vi "Case Next Frame.vi"(0 "Diagram in":refnum<vi>, 11 "error in (no error)":errorcluster) -> (4 "Selected Diagram":refnum<vi>, 6 "Selector":refnum<vi>, 8 "Inputs":refnum<vi>[](array[refnum]), 15 "error out":errorcluster)   [LabVIEW 2015, in "Scripting.lvlib"]
doc: "Navigates to the next frame of the Case Structure that owns <B>Diagram in</B>, supplying the frame's diagram at <B>Diagram out</B>. The input inside terminals and selector input terminal corresponding the diagram are output."
uses:
  Scripting.lvlib
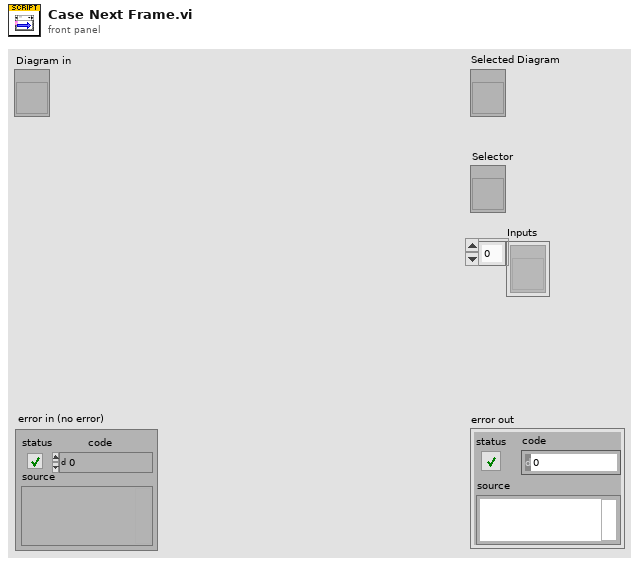
[diagram p1: front panel]
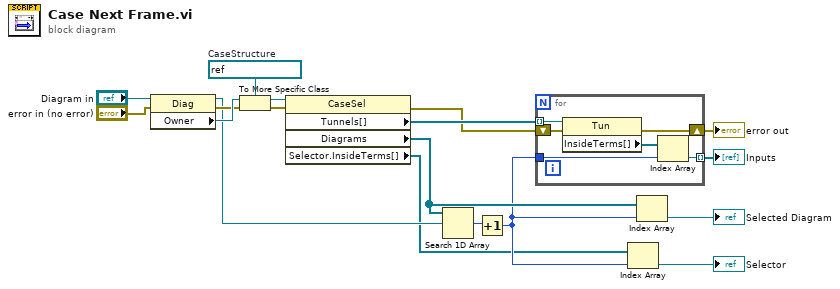
[diagram p0: block diagram]
diagram:
  w17 = refnum<vi> refnum  # CaseStructure
  n1 = property class="Diag"(reference="Diagram in", error in="error in (no error)") -> (reference out=w9:refnum<vi>, error out=w11:errorcluster, "Owner"=w12:refnum<vi>)
  n2 = To More Specific Class(target class=w17, reference=w12, error in=w11) -> (specific class reference=w3:refnum<vi>, error out=w2:errorcluster)
  n3 = property class="CaseSel"(reference=w3, error in=w2) -> (error out=w4:errorcluster, "Tunnels[]"=w5:refnum<vi>[], "Diagrams"=w8:refnum<vi>[], "Selector.InsideTerms[]"=w1:refnum<vi>[])  [unwired: 1 out]
  n4 = Search 1D Array(1D array=w8, element=w9) -> (index of element=w7:i32)  [unwired: 1 in]
  n5 = Increment(x=w7) -> (x+1=w6:i32)
  n6 = for {
    tunnel: w5 -> [w24] mode=indexing
    tunnel: w6 -> [w22]
    shift-right: [w20] -> w16
    shift-left: w4 -> [w21]
    tunnel: [w19] -> w15 mode=indexing
    n7 = property class="Tun"(reference=w24, error in=w21) -> (error out=w20:errorcluster, "InsideTerms[]"=w23:refnum<vi>[])  [unwired: 1 out]
    n8 = Index Array(array=w23, index=w22) -> (element=w19:refnum<vi>)
  }
  "error out" <- w16
  "Inputs" <- w15
  n9 = Index Array(array=w1, index=w6) -> (element=→"Selector":refnum<vi>)
  n10 = Index Array(array=w8, index=w6) -> (element=→"Selected Diagram":refnum<vi>)
